vi "Configure Demo Signal.vi"(7 "Enable Output (F: Disable)":bool, 8 "error in (no error)":errorcluster, 9 "Phase (90 degrees)":dbl=90.0, 10 "Demo Function (0: Sine)":i32(ring) items=["Sine", "Noise", "Phase", "Ringing", "Single", "AM", "Clock", "Glitch", "Burst", "MSO", "Runt", "Transition", "RF Burst", "Setup Hold", "LF Sine", "CAN", "LIN", "UART", "I2C", "SPI", "I2S", "CAN & LIN", "FM Burst", "ETE", "ARINC", "FlexRay", "MIL", "MIL2", "DC Motor", "SENT", "CFD", "Clock Jitter", "Real Time Eye", "Serial Data with Jitter"], 11 "VISA resource name":refnum<visa-resource-name>) -> (0 "error out":errorcluster, 3 "VISA resource name out":refnum<visa-resource-name>)   [LabVIEW 2016, in "Agilent 2000 3000 X-Series.lvlib"]
doc: "Configures the demo signal output."
uses:
  Agilent 2000 3000 X-Series.lvlib
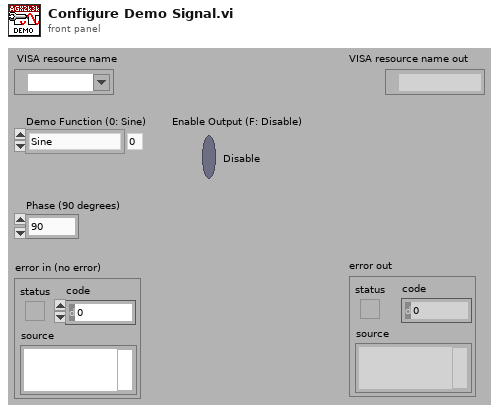
[diagram p1: front panel]
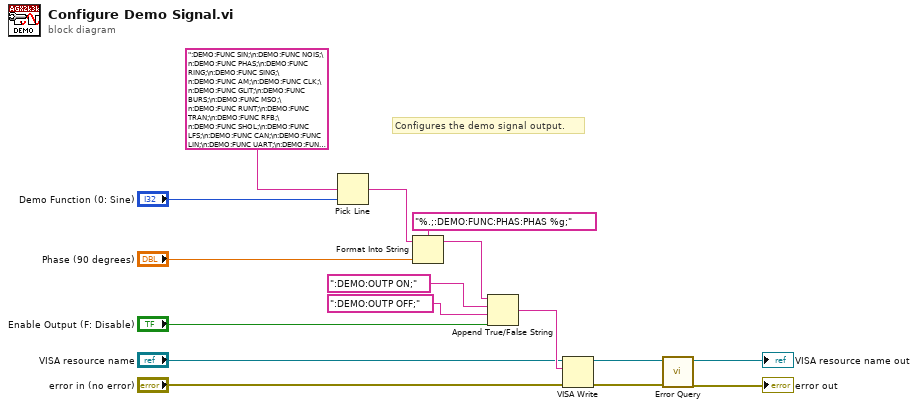
[diagram p0: block diagram]
diagram:
  # "Configures the demo signal output."
  n1 = Pick Line(multi-line string=":DEMO:FUNC SIN;\n:DEMO:FUNC NOIS;\n:DEMO:FUNC PHAS;\n:DEMO:FUNC RING;\n:DEMO:FUNC SING;\n:DEMO:FUNC AM;\n:DEMO:FUNC CLK;\n:DEMO:FUNC GLIT;\n:DEMO:FUNC BURS;\n:DEMO:FUNC MSO;\n:DEMO:FUNC RUNT;\n:DEMO:FUNC TRAN;\n:DEMO:FUNC RFB;\n:DEMO:FUNC SHOL;\n:DEMO:FUNC LFS;\n:DEMO:FUNC CAN;\n:DEMO:FUNC LIN;\n:DEMO:FUNC UART;\n:DEMO:FUNC I2C;\n:DEMO:FUNC SPI;\n:DEMO:FUNC I2S;\n:DEMO:FUNC CANL;\n:DEMO:FUNC FMB;\n:DEMO:FUNC ETE;\n:DEMO:FUNC ARIN;\n:DEMO:FUNC FLEX;\n:DEMO:FUNC MIL;\n:DEMO:FUNC MIL2;\n:DEMO:FUNC DCM;\n:DEMO:FUNC SENT;\n:DEMO:FUNC CFD;\n:DEMO:FUNC JITT;\n:DEMO:FUNC RTEY;\n:DEMO:FUNC SJIT;", line index="Demo Function (0: Sine)") -> (output string=w14:string)  [unwired: 1 out]
  n2 = Format Into String(format string="%.;:DEMO:FUNC:PHAS:PHAS %g;", initial string=w14, "Phase (90 degrees)") -> (resulting string=w11:string)  [unwired: 1 in, 1 out]
  n3 = Append True/False String(1:"Enable Output (F: Disable)", 2:":DEMO:OUTP OFF;", 3:":DEMO:OUTP ON;", 4:w11) -> (0:w7:string)
  n4 = VISA Write(VISA resource name="VISA resource name", write buffer=w7, error in (no error)="error in (no error)") -> (VISA resource name out=w4:refnum<visa-resource-name>, error out=w3:errorcluster)  [unwired: 1 out]
  n5 = call "Error Query.vi"("error in (no error)"=w3, "VISA resource name"=w4) -> ("error out"=→"error out":errorcluster, "VISA resource name out"=→"VISA resource name out":refnum<visa-resource-name>)  [unwired: 8 out]
